vi "产生随机方波.vi"() -> ()   [LabVIEW 2011]
panel:
  in  "频率随机产生":bool
  in  "幅值随机产生":bool
  out "波形图":dynamicdata(graph)
  in  "停止":bool
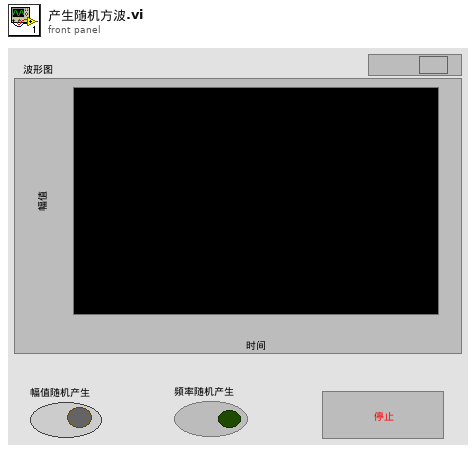
[diagram p1: front panel]
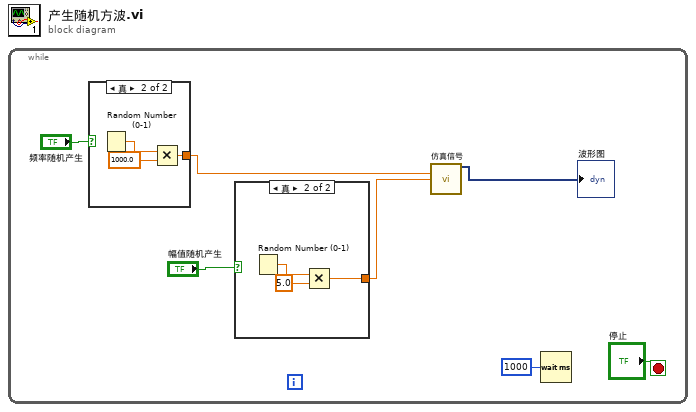
[diagram p0: block diagram]
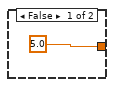
[diagram p2: hidden frame]
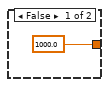
[diagram p3: hidden frame]
diagram:
  n1 = while {
    stop <- "停止" stop-if-true
    n2 = case shown="真" "频率随机产生" {
      tunnel: [1000.0 w13] -> w3
      frame False {
      }
      frame True {
        n3 = Random Number (0-1)() -> (number: 0 to 1=w14:dbl)
        n4 = Multiply(x=w14, y=1000.0) -> (x*y=w13:dbl)
      }
    }
    n5 = case shown="真" "幅值随机产生" {
      tunnel: [5.0 w9] -> w1
      frame False {
      }
      frame True {
        n6 = Random Number (0-1)() -> (number: 0 to 1=w11:dbl)
        n7 = Multiply(x=w11, y=5.0) -> (x*y=w9:dbl)
      }
    }
    n8 = call "仿真信号"("Frequency"=w3, "Amplitude"=w1) -> ("方波"=→"波形图":dynamicdata)  [unwired: 5 in, 8 out]
    n9 = Wait (ms)(milliseconds to wait=u32 1000 ("等待时间（毫秒）")) -> ()  [unwired: 1 out]
  }
